vi "Process PSD for Preview.vi"(7 "USRP Configuration":T1={"USRP RIO Resources"=["USRP-2945"], "LO Sharing"=TRUE, "Carrier Frequency (Hz)"=2000000000.0, "Gain"=40.0, "Sample rate (Hz)"=100000000.0, "reference frequency source"="Internal", "start trigger"=enum."Software"} {"Sample rate (Hz)" format="%#_6p"; "Carrier Frequency (Hz)" format="%#_6p"}, 8 "error in (no error)":errorcluster, 10 "Data Array":u64[](array[numeric]), 11 "Previewed Channel":T4) -> (0 "error out":errorcluster, 3 "Power Spectrum / PSD":cluster{"f0":dbl, "df":dbl, "magnitude":dbl[]})   [LabVIEW 2016]
uses:
  TDMS Raw to Channels/Previewed Channel - Enum.ctl
  TypeDefs/USRP Configuration.ctl
  <vilib>/userdefined/Silver/nirio_resource_slv.ctl
  29x5/SubVIs/Start Trigger.ctl
  <vilib>/measure/maspectr.llb/FFT Power Spectrum and PSD for 1 Chan (CDB).vi
  <vilib>/measure/NI_MAPro.lvlib
  <instrlib>/_niInstr/DSP/v1/FPGA/niInstr DSP v1 FPGA.lvlib
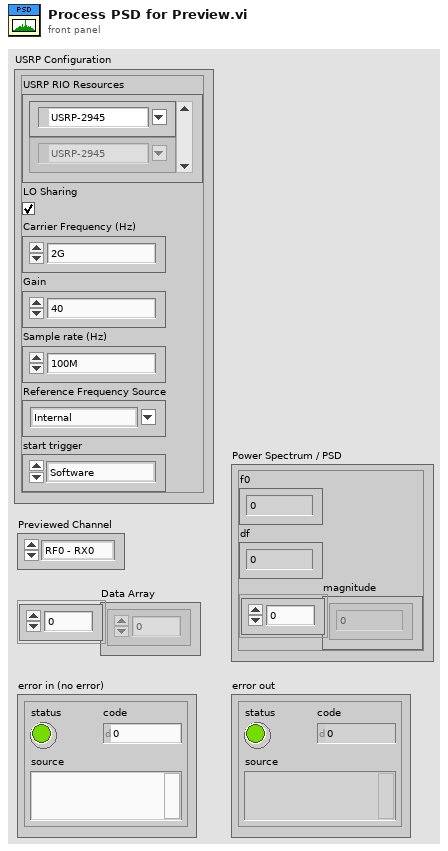
[diagram p1: front panel]
types:
  T1 = typedef "USRP Configuration.ctl" = cluster{"USRP RIO Resources":T2[], "LO Sharing":bool, "Carrier Frequency (Hz)":dbl, "Gain":dbl, "Sample rate (Hz)":dbl, "reference frequency source":string, "start trigger":T3}
  T2 = typedef "nirio_resource_slv.ctl" = tag
  T3 = typedef "Start Trigger.ctl" = enum8{"Software", "Digital Edge", "Rx Start Trigger", "Tx Start Trigger", "Immediate", "Future Time Event"}
  T4 = typedef "Previewed Channel - Enum.ctl" = enum16{"RF0 - RX0", "RF0 - RX1", "RF1 - RX0", "RF1 - RX1"}
  T5 = typedef "niInstr DSP v1 Shared.lvlib/IQ Data.ctl" = cluster{"I":fxp<+/-,18,1>, "Q":fxp<+/-,18,1>, "overflow":bool}
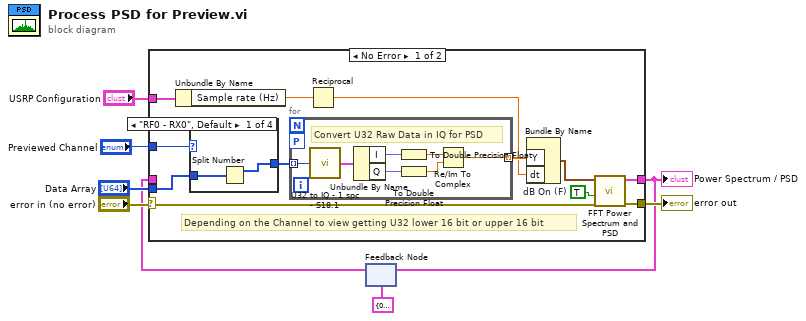
[diagram p0: block diagram]
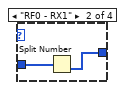
[diagram p2: hidden frame]
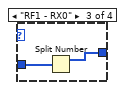
[diagram p3: hidden frame]
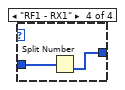
[diagram p4: hidden frame]
diagram:
  n1 = feedback #1(cluster{"f0":dbl, "df":dbl, "magnitude":dbl[]} {"f0"=0.0, "df"=0.0, "magnitude"=[]} ("Power Spectrum / PSD")) -> (w2:cluster{"f0":dbl, "df":dbl, "magnitude":dbl[]})
  n2 = case shown="No Error" "error in (no error)" {
    selector: "error in (no error)" -> [w14 w37]
    tunnel: "Data Array" -> [w20 _]
    tunnel: "Previewed Channel" -> [w19 _]
    tunnel: [w16 w36] -> w3
    tunnel: [w15 w37] -> w6
    tunnel: "USRP Configuration" -> [w10 _]
    tunnel: w2 -> [_ w36]
    frame No Error {
      w18 = TRUE  # dB On (F)
      # "Depending on the Channel to view getting U32 lower 16 bit or upper 16 bit"
      n3 = Unbundle By Name(w10) -> ("Sample rate (Hz)"=w9:dbl)
      n4 = case shown="\"RF0 - RX0\", Default" w19 {
        tunnel: [w29 w31 w33 w35] -> w13
        tunnel: w20 -> [w28 w30 w32 w34]
        frame "RF0 - RX0", Default {
          n5 = Split Number(x=w28) -> (hi(x)=w29:u32[])  [unwired: 1 out]
        }
        frame "RF0 - RX1" {
          n6 = Split Number(x=w30) -> (lo(x)=w31:u32[])  [unwired: 1 out]
        }
        frame "RF1 - RX0" {
          n7 = Split Number(x=w32) -> (hi(x)=w33:u32[])  [unwired: 1 out]
        }
        frame "RF1 - RX1" {
          n8 = Split Number(x=w34) -> (lo(x)=w35:u32[])  [unwired: 1 out]
        }
      }
      n9 = for {
        tunnel: w13 -> [w27] mode=indexing
        tunnel: [w21] -> w12 mode=indexing
        workers-P: _ -> [_]
        # "Convert U32 Raw Data in IQ for PSD"
        n10 = call <instrlib>:"U32 to IQ - 1 spc - S18.1.vi"("U32 data"=w27) -> ("IQ data"=w22:T5)  [unwired: 14 in]
        n11 = Unbundle By Name(w22) -> ("I"=w24:fxp<+/-,18,1>, "Q"=w25:fxp<+/-,18,1>)
        n12 = To Double Precision Float(number=w24) -> (double precision float=w23:dbl)
        n13 = To Double Precision Float(number=w25) -> (double precision float=w26:dbl)
        n14 = Re/Im To Complex(1:w26, 2:w23) -> (0:w21:cdb)
      }
      n15 = Reciprocal(x=w9) -> (1/x=w11:dbl)
      n16 = Bundle By Name("Y"=w12, "dt"=w11) -> (w17:waveform(cdb))  [unwired: 1 in]
      n17 = call-poly <vilib>:"FFT Power Spectrum and PSD.vi"("error in (no error)"=w14, "dB On (F)"=w18, "time signal"=w17) -> ("error out"=w15:errorcluster, "Power Spectrum / PSD"=w16:cluster{"f0":dbl, "df":dbl, "magnitude":dbl[]})  [unwired: 5 in, 2 out]
    }
    frame Error {
    }
  }
  "Power Spectrum / PSD" <- w3
  "error out" <- w6
  n18 = feedback-in #1(w3) -> ()
